vi "Record Call.vi"(8 "error in (no error)":errorcluster, 10 "VI Call":refnum<class "VI Call.lvclass">, 11 "Expectation in":refnum<class "Expectation.lvclass">) -> (0 "error out":errorcluster, 3 "Expectation out":refnum<class "Expectation.lvclass">)   [LabVIEW 2020, in "Expectation.lvclass"]
uses:
  Expectation.lvclass
  VI Call/VI Call.lvclass
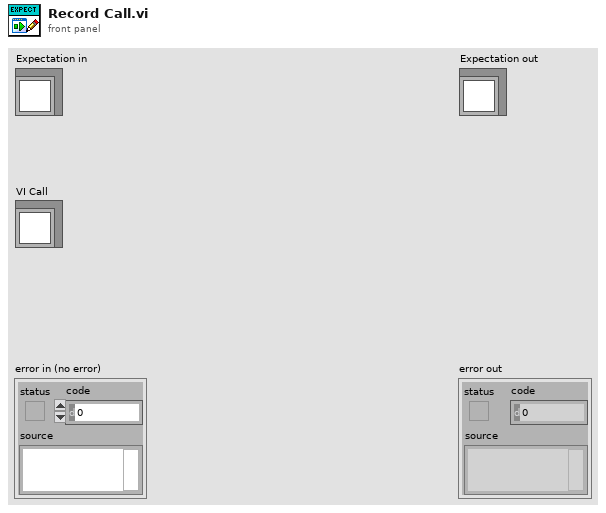
[diagram p1: front panel]
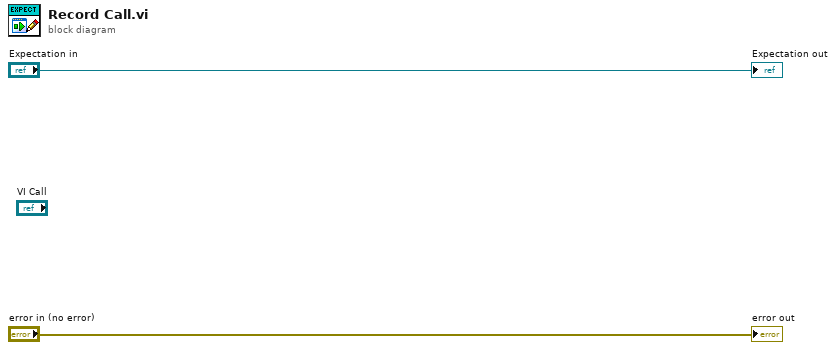
[diagram p0: block diagram]
diagram:
  "error out" <- "error in (no error)"
  "Expectation out" <- "Expectation in"
